vi "IP2SVName.vi"() -> (10 "name":string)   [LabVIEW 2009, in "MoAgSy.lvlib"]
uses:
  MoAgSy.lvlib
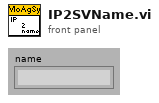
[diagram p1: front panel]
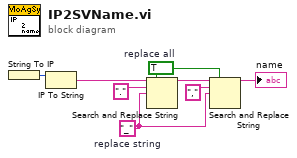
[diagram p0: block diagram]
diagram:
  w2 = "_"  # replace string
  w3 = TRUE  # replace all
  n1 = String To IP() -> (0:w8:u32)  [unwired: 1 in]
  n2 = IP To String(2:w8) -> (0:w7:string)  [unwired: 1 in]
  n3 = Search and Replace String(replace all?=w3, input string=w7, search string=".", replace string=w2) -> (result string=w5:string)  [unwired: 4 in, 3 out]
  n4 = Search and Replace String(replace all?=w3, input string=w5, search string=",", replace string=w2) -> (result string=→"name":string)  [unwired: 4 in, 3 out]
